vi "FGV Frontpanel Position CG.vi"(0 "Dieses VI":refnum<vi>, 11 "error in (no error)":errorcluster caption="Fehler (Eingang, kein Fehler)", 13 "Aktion":T2) -> (4 "Front Panel.WinBounds":T1, 8 "Bit":bool, 15 "error out":errorcluster caption="Fehler (Ausgang)")   [LabVIEW 2020, in "CalGas Aufschaltung.lvlib"]
uses:
  CalGas Aufschaltung.lvlib
  FGV Frontpanel Position CG.ctl
  <vilib>/Utility/miscctls.llb/LVRectTypeDef.ctl
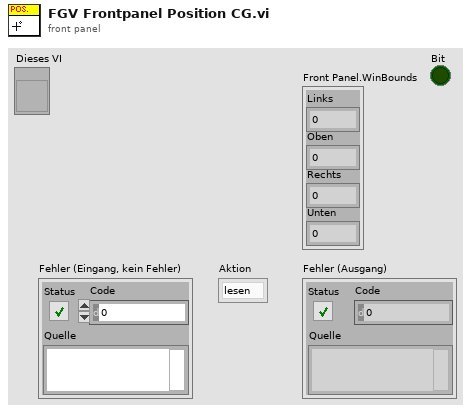
[diagram p1: front panel]
types:
  T1 = typedef "LVRectTypeDef.ctl" = cluster{"Left":i16, "Top":i16, "Right":i16, "Bottom":i16}
  T2 = typedef "CalGas Aufschaltung.lvlib/FGV Frontpanel Position CG.ctl" = enum16{"lesen", "init", "Position speichern", "bit löschen"}
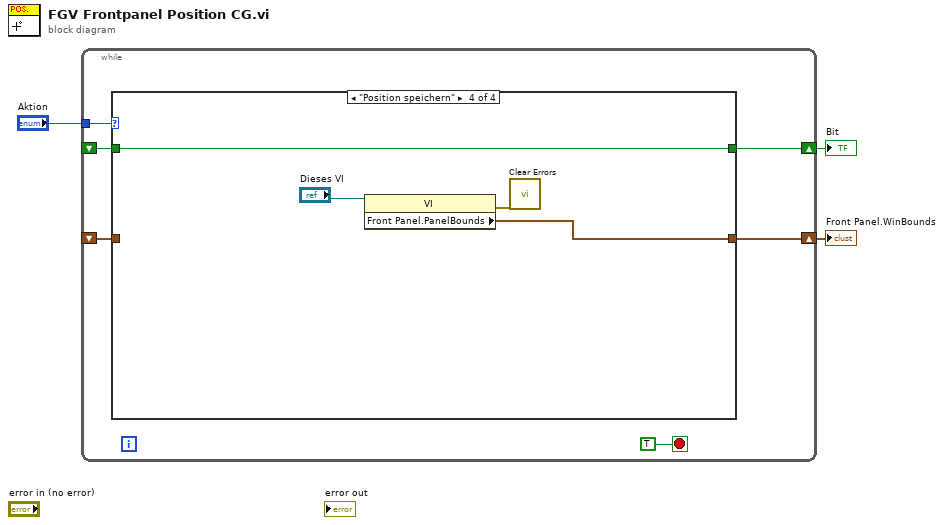
[diagram p0: block diagram]
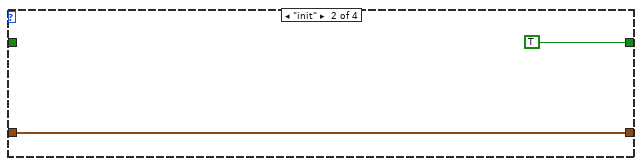
[diagram p3: hidden frame]
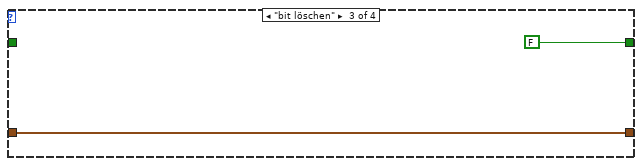
[diagram p4: hidden frame]
diagram:
  n1 = while {
    tunnel: "Aktion" -> [w8]
    shift-right: [w7] -> w2
    shift-left: _ -> [w6]
    shift-right: [w5] -> w1
    shift-left: _ -> [w4]
    stop <- TRUE stop-if-true
    n2 = case shown="\"Position speichern\"" w8 {
      tunnel: [w11 w13 w15 w17] -> w7
      tunnel: w6 -> [w11 w13 w15 _]
      tunnel: [w10 TRUE FALSE w19] -> w5
      tunnel: w4 -> [w10 _ _ w19]
      frame "lesen", Default {
      }
      frame "init" {
      }
      frame "bit löschen" {
      }
      frame "Position speichern" {
        n3 = property class="VI"(reference="Dieses VI") -> (error out=w16:errorcluster, "Front Panel.PanelBounds"=w17:T1)  [unwired: 1 in, 1 out]
        n4 = call <vilib>:"Clear Errors.vi"("error in (no error)"=w16) -> ()  [unwired: 5 in, 2 out]
      }
    }
  }
  "Front Panel.WinBounds" <- w2
  "Bit" <- w1
